vi "Flatten and Save Class Data.vi"(8 "error in":errorcluster, 11 "Loopback in":refnum<class "Loopback.lvclass">) -> (0 "error out":errorcluster, 3 "Loopback out":refnum<class "Loopback.lvclass">)   [LabVIEW 2020, in "Loopback.lvclass"]
uses:
  Loopback.lvclass
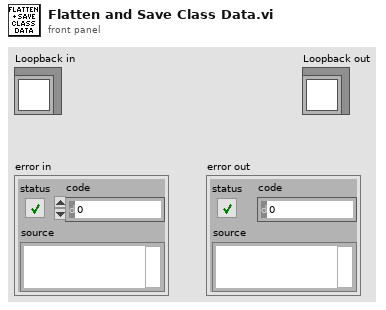
[diagram p1: front panel]
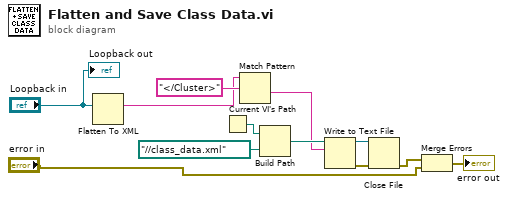
[diagram p0: block diagram]
diagram:
  n1 = Flatten To XML(6:"Loopback in") -> (2:w5:string)
  n2 = Current VI's Path() -> (path=w9:path)
  n3 = Match Pattern(string=w5, regular expression="</Cluster>") -> (after substring=w4:string)  [unwired: 1 in, 3 out]
  n4 = Build Path(base path=w9, name or relative path=path "../../class_data.xml") -> (appended path=w11:path)
  n5 = Write to Text File(file (use dialog)=w11, text=w4) -> (refnum out=w7:refnum<file>, error out=w12:errorcluster)  [unwired: 2 in, 1 out]
  n6 = Close File(refnum=w7, error in=w12) -> (error out=w3:errorcluster)  [unwired: 1 out]
  n7 = Merge Errors(w3, "error in") -> (→"error out":errorcluster)
  "Loopback out" <- "Loopback in"
